vi "check_styx_err.vi"(8 "error in (no error)":errorcluster, 9 "Additional Comment":string, 10 "return val":i32) -> (0 "error out":errorcluster)   [LabVIEW 2010, in "lib1299.lvlib"]
uses:
  lib1299.lvlib
  cstyx/win32/cstyx.dll
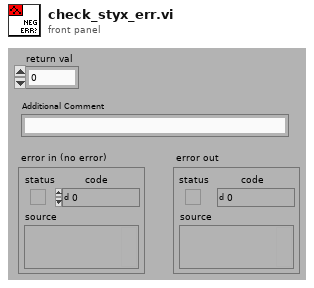
[diagram p1: front panel]
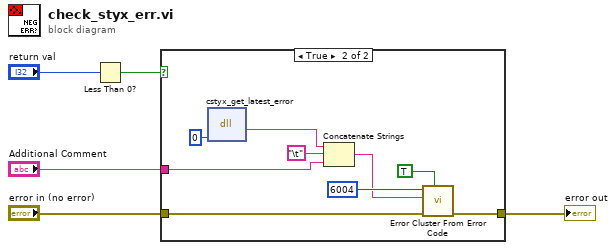
[diagram p0: block diagram]
diagram:
  n1 = Less Than 0?(x="return val") -> (x < 0?=w3:bool)
  n2 = case shown="True" w3 {
    tunnel: [w6 w12] -> w5
    tunnel: "error in (no error)" -> [w6 w13]
    tunnel: "Additional Comment" -> [_ w9]
    frame False {
    }
    frame True {
      n3 = dll-call lib="C:/work/ads1299evm/lib_1299/Styx/cstyx/win32/cstyx.dll" fn="cstyx_get_latest_error"("code"=0) -> (w10:string)  [unwired: 4 in, 2 out]
      n4 = Concatenate Strings(w10, "\t", w9) -> (w8:string)
      n5 = call <vilib>:"Error Cluster From Error Code.vi"("show call chain? (False)"=TRUE, "error in (no error)"=w13, "error message (\"\")"=w8, "error code (0)"=6004 ("[error code] (0)")) -> ("error out"=w12:errorcluster)  [unwired: 5 in]
    }
  }
  "error out" <- w5
